vi "FindAllMessages.vi"(8 "error in (no error)":errorcluster, 11 "CS++MessageMakerMain in":refnum<class "CS++MessageMakerMain.lvclass">) -> (0 "error out":errorcluster, 3 "CS++MessageMakerMain out":refnum<class "CS++MessageMakerMain.lvclass">)   [LabVIEW 2014, in "CS++MessageMakerMain.lvlib" / "CS++MessageMakerMain.lvclass"]
doc: "Search for all Messages in a project. Needed during the Initilaization procedure."
uses:
  CS++MessageMakerMain.lvclass
  CS++MessageMakerMain.lvclass/CS++MessageMakerMain.ctl
  CSPP_Actor/CS++Actor.lvclass
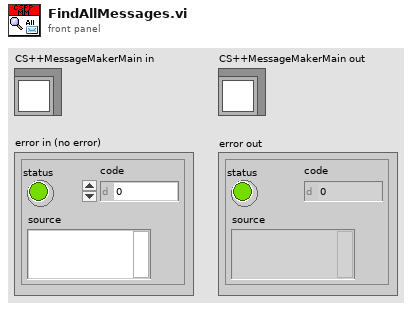
[diagram p1: front panel]
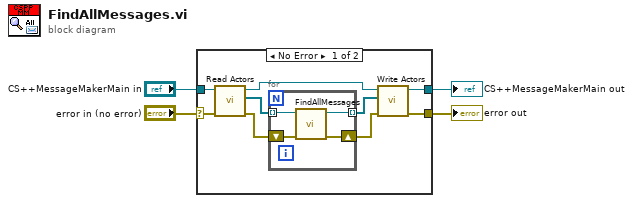
[diagram p0: block diagram]
diagram:
  n1 = case shown="No Error" "error in (no error)" {
    selector: "error in (no error)" -> [w12 w19]
    tunnel: [w6 w19] -> w3
    tunnel: [w5 w18] -> w1
    tunnel: "CS++MessageMakerMain in" -> [w13 w18]
    frame No Error {
      n2 = call "Read Actors.vi"("error in (no error)"=w12, "CS++MessageMakerMain in"=w13) -> ("error out"=w10:errorcluster, "Actors"=w11:refnum<class "CS++Actor.lvclass">[], "CS++MessageMakerMain out"=w7:refnum<class "CS++MessageMakerMain.lvclass">)  [unwired: 7 in]
      n3 = for {
        tunnel: w11 -> [w17] mode=indexing
        shift-right: [w15] -> w9
        shift-left: w10 -> [w16]
        tunnel: [w14] -> w8 mode=indexing
        n4 = call "FindAllMessages.vi"("error in (no error)"=w16, "CS++Actor in"=w17) -> ("error out"=w15:errorcluster, "CS++Actor out"=w14:refnum<class "CS++Actor.lvclass">)  [unwired: 8 in]
      }
      n5 = call "Write Actors.vi"("error in (no error)"=w9, "Actors"=w8, "CS++MessageMakerMain in"=w7) -> ("error out"=w6:errorcluster, "CS++MessageMakerMain out"=w5:refnum<class "CS++MessageMakerMain.lvclass">)  [unwired: 7 in]
    }
    frame Error {
    }
  }
  "error out" <- w3
  "CS++MessageMakerMain out" <- w1
